vi "Calculator.vi"() -> ()   [LabVIEW 2020]
panel:
  in  "error in (no error)":errorcluster
  out "error out":errorcluster
  out "ANSWER":string
  in  "Cluster":T1
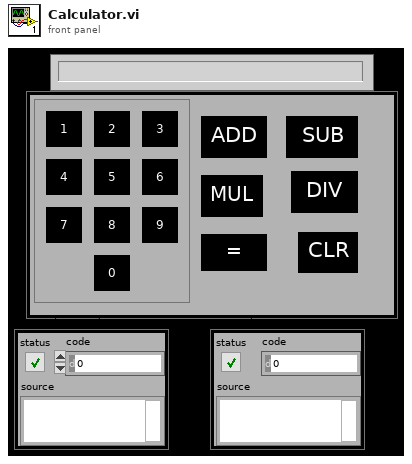
[diagram p1: front panel]
types:
  T1 = cluster{"1":bool, "2":bool, " 3":bool, " 4":bool, " 5":bool, " 6":bool, " 7":bool, " 8":bool, " 9":bool, " 0":bool, "ADD":bool, "SUB":bool, "DIV":bool, "EQUAL":bool, "CLEAR":bool, "MUL":bool}
  T2 = enum16{"Nofunc", "ADD", "SUB", "MUL", "DIV", "SQR", "SQRT"}
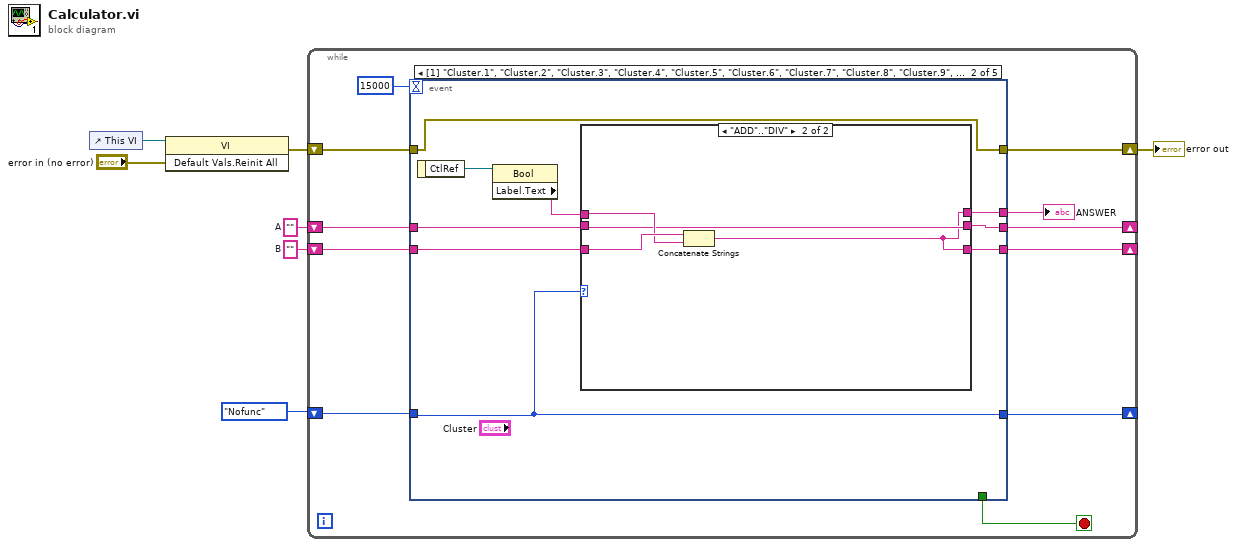
[diagram p0: block diagram]
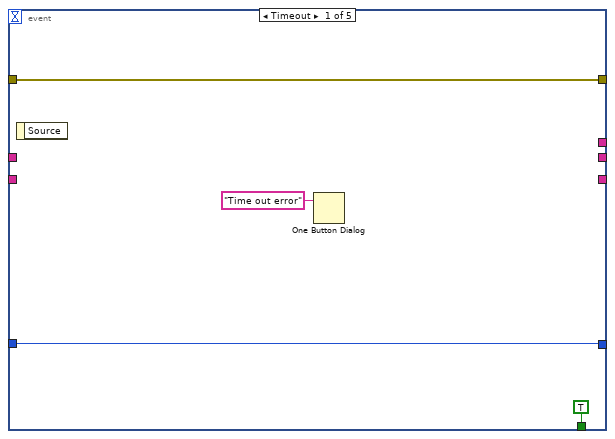
[diagram p2: hidden frame]
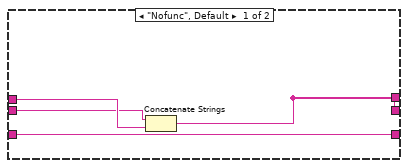
[diagram p3: hidden frame]
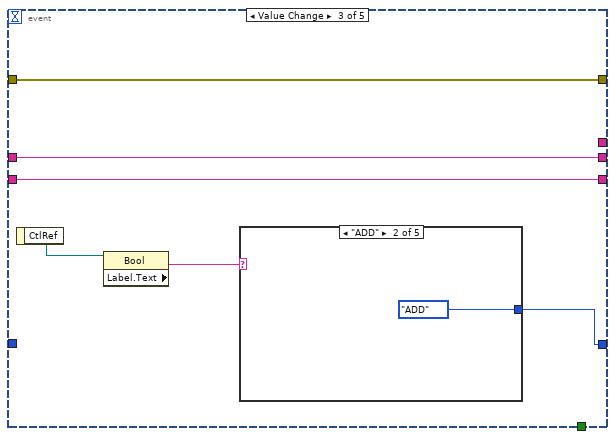
[diagram p4: hidden frame]
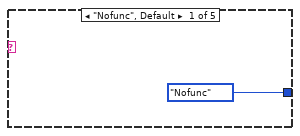
[diagram p5: hidden frame]
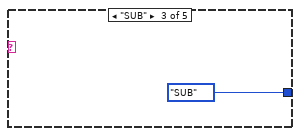
[diagram p6: hidden frame]
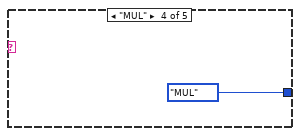
[diagram p7: hidden frame]
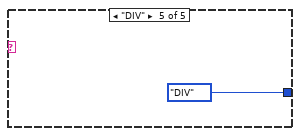
[diagram p8: hidden frame]
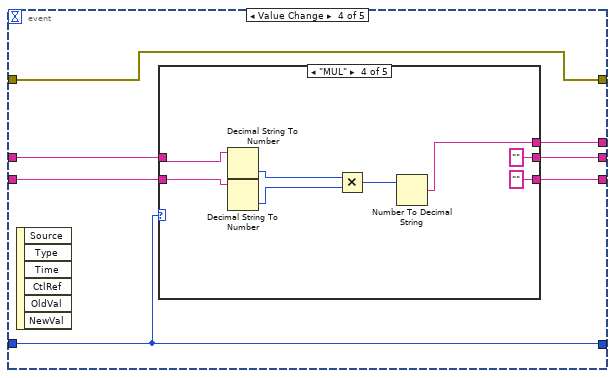
[diagram p9: hidden frame]
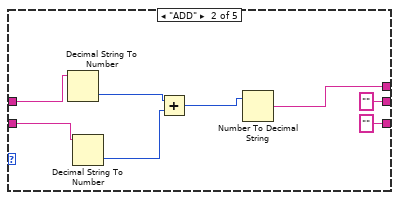
[diagram p11: hidden frame]
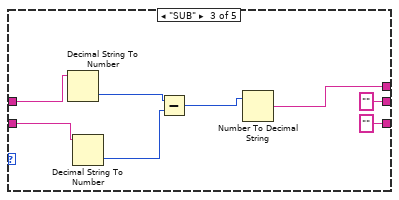
[diagram p12: hidden frame]
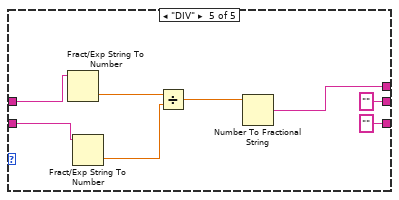
[diagram p13: hidden frame]
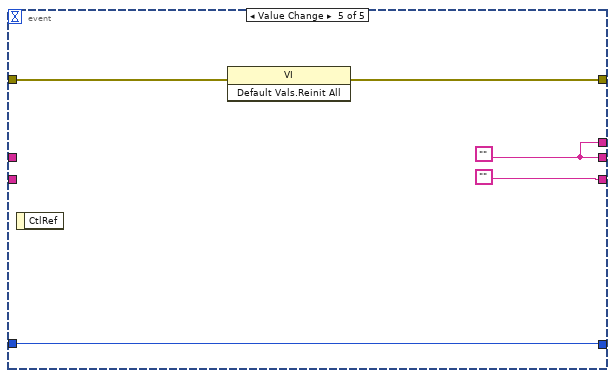
[diagram p14: hidden frame]
diagram:
  w6 = ""  # B
  w7 = ""  # A
  n1 = control-ref of="This VI"() -> (w4:refnum<vi>)
  n2 = invoke class="VI" method="Default Vals.Reinit All"(reference=w4, error in="error in (no error)") -> (error out=w3:errorcluster)  [unwired: 1 in, 2 out]
  n3 = while {
    shift-right: [w14] -> _
    shift-left: w7 -> [w17]
    shift-right: [w15] -> _
    shift-left: w6 -> [w16]
    shift-right: [w12] -> _
    shift-left: enum16{"Nofunc", "ADD", "SUB", "MUL", "DIV"}."Nofunc" -> [w8]
    shift-right: [w9] -> w2
    shift-left: w3 -> [w10]
    stop <- w11 stop-if-true
    n4 = event shown="[1] \"Cluster.1\", \"Cluster.2\", \"Cluster.3\", \"Cluster.4\", \"Cluster.5\", \"Cluster.6\", \"Cluster.7\", \"Cluster.8\", \"Cluster.9\", \"Cluster.0\": Value Change" {
      selector: _ -> [_ _ _ _ _]
      dyn-events: _ -> [_ _ _ _ _]
      timeout: 15000 -> [_ _ _ _ _]
      tunnel: w17 -> [_ w29 w44 w56 _]
      tunnel: w16 -> [_ w28 w43 w54 _]
      tunnel: w8 -> [w22 w27 _ w57 w96]
      tunnel: [w22 w27 w41 w57 w96] -> w12
      tunnel: [_ w26 w43 w53 ""] -> w15
      tunnel: [_ w25 w44 w55 w92] -> w14
      tunnel: [_ w24 _ w52 w92] -> w13
      tunnel: [TRUE ("stop") _ _ _ _] -> w11
      tunnel: w10 -> [w19 w23 w40 w51 w95]
      tunnel: [w19 w23 w40 w51 w94] -> w9
      event Timeout {
        n5 = event-data() -> ()  [unwired: 1 in, 1 out]
        n6 = One Button Dialog(message="Time out error") -> ()  [unwired: 1 in, 1 out]
      }
      event "Cluster.1", "Cluster.2", "Cluster.3", "Cluster.4", "Cluster.5", "Cluster.6", "Cluster.7", "Cluster.8", "Cluster.9", "Cluster.0": Value Change {
        n7 = event-data() -> ("CtlRef"=w31:refnum<vi>)  [unwired: 1 in]
        n8 = property class="Bool"(reference=w31) -> ("Label.Text"=w30:string)  [unwired: 1 in, 2 out]
        n9 = case shown="\"ADD\"..\"DIV\"" w27 {
          tunnel: w30 -> [w35 w38]
          tunnel: w29 -> [w34 w37]
          tunnel: w28 -> [w32 w39]
          tunnel: [w32 w36] -> w26
          tunnel: [w33 w37] -> w25
          tunnel: [w33 w36] -> w24
          frame "Nofunc", Default {
            n10 = Concatenate Strings(w34, w35) -> (w33:string)
          }
          frame "ADD".."DIV" {
            n11 = Concatenate Strings(w39, w38) -> (w36:string)
          }
        }
      }
      event "Cluster.ADD", "Cluster.SUB", "Cluster.MUL", "Cluster.DIV": Value Change {
        n12 = event-data() -> ("CtlRef"=w45:refnum<vi>)  [unwired: 1 in]
        n13 = property class="Bool"(reference=w45) -> ("Label.Text"=w42:string)  [unwired: 1 in, 2 out]
        n14 = case shown="\"ADD\"" w42 {
          tunnel: [T2."Nofunc" T2."ADD" T2."SUB" T2."MUL" T2."DIV"] -> w41
          frame "Nofunc", Default {
          }
          frame "ADD" {
          }
          frame "SUB" {
          }
          frame "MUL" {
          }
          frame "DIV" {
          }
        }
      }
      event "Cluster.EQUAL": Value Change {
        n15 = event-data() -> ()  [unwired: 1 in, 6 out]
        n16 = case shown="\"MUL\"" w57 {
          tunnel: w56 -> [w58 w67 w75 w83 w91]
          tunnel: [w58 "" ("A") "" ("A") "" ("A") "" ("A")] -> w55
          tunnel: w54 -> [w59 w66 w74 w82 w90]
          tunnel: [w59 "" ("B") "" ("B") "" ("B") "" ("B")] -> w53
          tunnel: [w58 w62 w70 w78 w86] -> w52
          frame "Nofunc", Default {
          }
          frame "ADD" {
            n17 = Decimal String To Number(string=w67) -> (number=w65:i32)  [unwired: 2 in, 1 out]
            n18 = Decimal String To Number(string=w66) -> (number=w64:i32)  [unwired: 2 in, 1 out]
            n19 = Add(x=w65, y=w64) -> (x+y=w63:i32)
            n20 = Number To Decimal String(number=w63) -> (decimal integer string=w62:string)  [unwired: 1 in]
          }
          frame "SUB" {
            n21 = Decimal String To Number(string=w75) -> (number=w73:i32)  [unwired: 2 in, 1 out]
            n22 = Decimal String To Number(string=w74) -> (number=w72:i32)  [unwired: 2 in, 1 out]
            n23 = Subtract(x=w73, y=w72) -> (x-y=w71:i32)
            n24 = Number To Decimal String(number=w71) -> (decimal integer string=w70:string)  [unwired: 1 in]
          }
          frame "MUL" {
            n25 = Decimal String To Number(string=w83) -> (number=w81:i32)  [unwired: 2 in, 1 out]
            n26 = Decimal String To Number(string=w82) -> (number=w80:i32)  [unwired: 2 in, 1 out]
            n27 = Multiply(x=w81, y=w80) -> (x*y=w79:i32)
            n28 = Number To Decimal String(number=w79) -> (decimal integer string=w78:string)  [unwired: 1 in]
          }
          frame "DIV" {
            n29 = Fract/Exp String To Number(string=w91) -> (number=w89:dbl)  [unwired: 3 in, 1 out]
            n30 = Fract/Exp String To Number(string=w90) -> (number=w88:dbl)  [unwired: 3 in, 1 out]
            n31 = Divide(x=w89, y=w88) -> (x/y=w87:dbl)
            n32 = Number To Fractional String(number=w87) -> (F-format string=w86:string)  [unwired: 3 in]
          }
        }
      }
      event "Cluster.CLEAR": Value Change {
        w92 = ""
        n33 = event-data() -> ()  [unwired: 1 in, 1 out]
        n34 = invoke class="VI" method="Default Vals.Reinit All"(error in=w95) -> (error out=w94:errorcluster)  [unwired: 2 in, 2 out]
      }
    }
    "ANSWER" <- w13
  }
  "error out" <- w2
